vi "LoadNodeUI.vi"(7 "user event out":T1, 8 "error in":errorcluster, 9 "sub panel ref in":refnum<vi>, 10 "main queue":T3, 11 "node":T2) -> (0 "error out":errorcluster)   [LabVIEW 2013, in "NISE_CEF_TreeControl.lvlib"]
doc: "This VI will insert the UI from a node into a subpanel."
uses:
  NISE_CEF_TreeControl.lvlib
  <vilib>/NI/AMC/Message Queue.ctl
  <vilib>/NI/AMC/Message.ctl
  <vilib>/NI/Tools/Keyed Array/KeyedArray.ctl
  Node/NodeRef.ctl
  Node/NISE_CEF_Node.lvclass
  Node/UserEventRef.ctl
  Controls/EventCluster.ctl
  <vilib>/NI/Tools/Keyed Array/Tools_KeyedArray.lvlib
  <vilib>/NI/AMC/AMC.lvlib
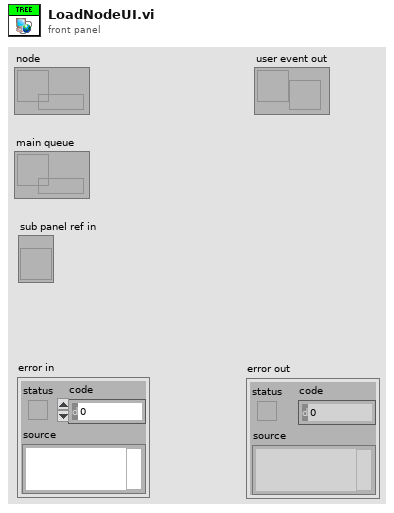
[diagram p1: front panel]
types:
  T1 = typedef "NISE_CEF_Node.lvclass/UserEventRef.ctl" = refnum<user-event>
  T2 = typedef "NISE_CEF_Node.lvclass/NodeRef.ctl" = refnum<data-value>
  T3 = typedef "AMC.lvlib/Message Queue.ctl" = refnum<queue>
  T4 = enum32{"Bad", "Idle", "Run top level", "Running"}
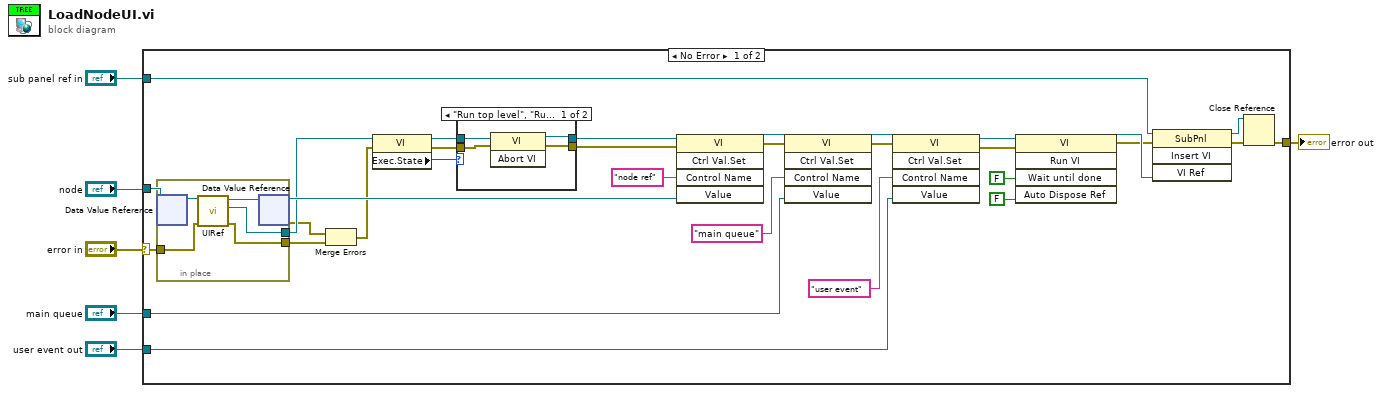
[diagram p0: block diagram]
diagram:
  n1 = case shown="No Error" "error in" {
    selector: "error in" -> [w20 w49]
    tunnel: [w27 w49] -> w5
    tunnel: "node" -> [w13 _]
    tunnel: "main queue" -> [w12 _]
    tunnel: "user event out" -> [w11 _]
    tunnel: "sub panel ref in" -> [w10 _]
    frame No Error {
      n2 = in-place {
        in-place-border: w20 -> [w45]
        in-place-border: [w46] -> w19
        in-place-border: [w44] -> w9
        n3 = in-place-dvr #1(w13) -> (w48:refnum<class "NISE_CEF_Node.lvclass">)  [unwired: 1 out]
        n4 = call-dynamic "UIRef.vi"("error in"=w45, "node in"=w48) -> ("error out"=w44:errorcluster, "VI refnum"=w46:refnum<vi>, "node out"=w47:refnum<class "NISE_CEF_Node.lvclass">)  [unwired: 7 in]
        n5 = in-place-dvr #1(w47) -> (w21:T2, w8:errorcluster)
      }
      n6 = Merge Errors(w8, w9) -> (w7:errorcluster)
      n7 = property class="VI"(reference=w19, error in=w7) -> (reference out=w16:refnum<vi>, error out=w15:errorcluster, "Exec.State"=w18:T4)
      n8 = case shown="\"Run top level\", \"Running\"" w18 {
        tunnel: [w38 w43] -> w17
        tunnel: w16 -> [w41 w43]
        tunnel: w15 -> [w40 w42]
        tunnel: [w39 w42] -> w14
        frame "Run top level", "Running" {
          n9 = invoke class="VI" method="Abort VI"(reference=w41, error in=w40) -> (reference out=w38:refnum<vi>, error out=w39:errorcluster)  [unwired: 1 in, 1 out]
        }
        frame "Idle", Default {
        }
      }
      n10 = invoke class="VI" method="Ctrl Val.Set"(reference=w17, error in=w14, "Control Name"="node ref", "Value"=w21) -> (reference out=w35:refnum<vi>, error out=w30:errorcluster)  [unwired: 1 in, 3 out]
      n11 = invoke class="VI" method="Ctrl Val.Set"(reference=w35, error in=w30, "Control Name"="main queue", "Value"=w12) -> (reference out=w25:refnum<vi>, error out=w26:errorcluster)  [unwired: 1 in, 3 out]
      n12 = invoke class="VI" method="Ctrl Val.Set"(reference=w25, error in=w26, "Control Name"="user event", "Value"=w11) -> (reference out=w24:refnum<vi>, error out=w23:errorcluster)  [unwired: 1 in, 3 out]
      n13 = invoke class="VI" method="Run VI"(reference=w24, error in=w23, "Wait until done"=FALSE ("Wait Until Done"), "Auto Dispose Ref"=FALSE ("Auto Dispose Reference")) -> (reference out=w34:refnum<vi>, error out=w33:errorcluster)  [unwired: 1 in, 3 out]
      n14 = invoke class="SubPnl" method="Insert VI"(reference=w10, error in=w33, "VI Ref"=w34) -> (reference out=w28:refnum<vi>, error out=w29:errorcluster)  [unwired: 1 in, 2 out]
      n15 = Close Reference(reference=w28, error in (no error)=w29) -> (error out=w27:errorcluster)
    }
    frame Error {
    }
  }
  "error out" <- w5
